vi "ActorRefContainer Write Modules.vi"(8 "error in (no error)":errorcluster, 10 "Modules":T1, 11 "ActorRefContainer in":refnum<class "ActorRefContainer.lvclass">) -> (0 "error out":errorcluster, 3 "ActorRefContainer out":refnum<class "ActorRefContainer.lvclass">)   [LabVIEW 2019, in "ActorRefContainer.lvlib" / "ActorRefContainer.lvclass"]
uses:
  ActorRefContainer.lvclass
  TypeDef/Active Modules REF.ctl
  <vilib>/ActorFramework/Message Enqueuer/Message Enqueuer.lvclass
  ActorRefContainer.lvclass/ActorRefContainer.ctl
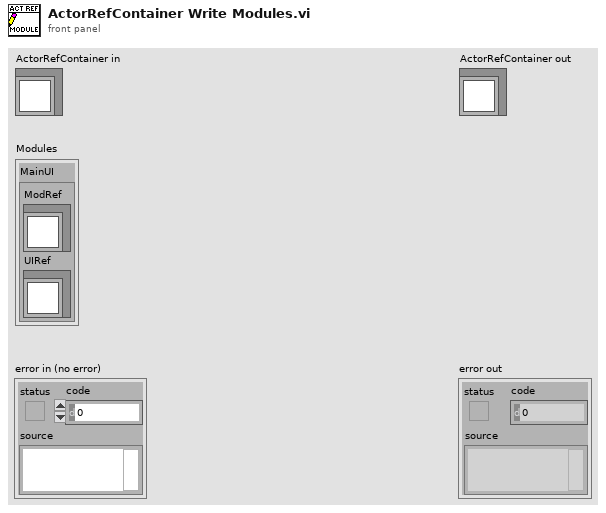
[diagram p1: front panel]
types:
  T1 = typedef "ActorRefContainer.lvlib/ActorRefContainer.lvclass/Active Modules REF.ctl" = cluster{"MainUI":cluster{"ModRef":refnum<class "Message Enqueuer.lvclass">, "UIRef":refnum<class "Message Enqueuer.lvclass">}}
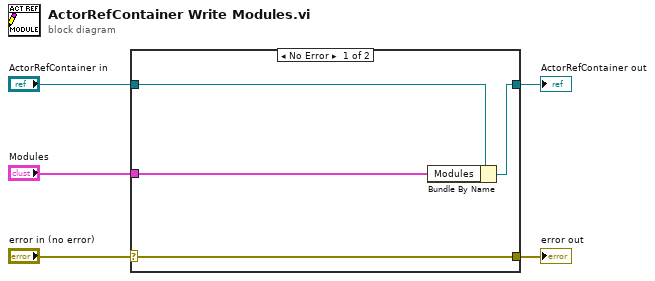
[diagram p0: block diagram]
diagram:
  n1 = case shown="No Error" "error in (no error)" {
    selector: "error in (no error)" -> [w9 w10]
    tunnel: [w9 w10] -> w4
    tunnel: [w7 w11] -> w2
    tunnel: "ActorRefContainer in" -> [w8 w11]
    tunnel: "Modules" -> [w6 _]
    frame No Error {
      n2 = Bundle By Name(cluster=w8, "Modules"=w6) -> (w7:refnum<class "ActorRefContainer.lvclass">)
    }
    frame Error {
    }
  }
  "error out" <- w4
  "ActorRefContainer out" <- w2
